vi "SRV_Build Video Stream Rate Command.vi"(10 "Video Stream Rate Period (ms)":u32) -> (1 "Command String":string, 2 "Command Array":u8[](array[numeric]) format="%.0b")   [LabVIEW 2014]
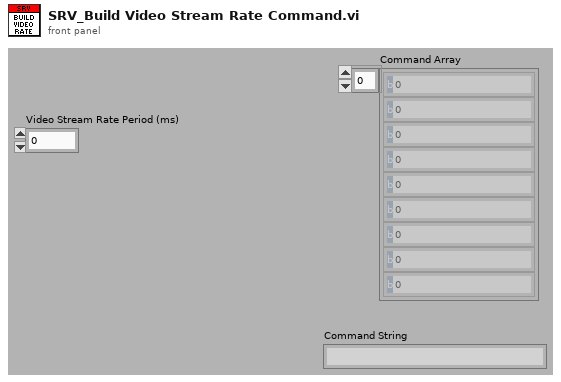
[diagram p1: front panel]
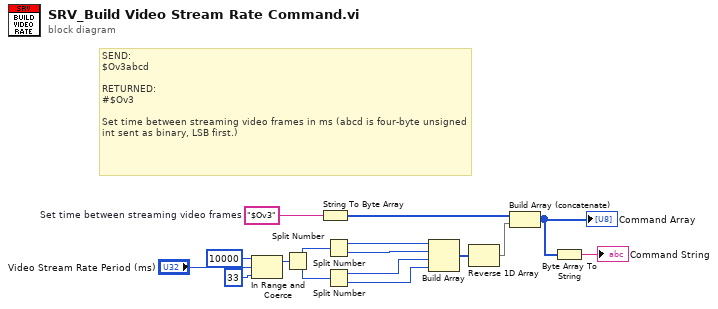
[diagram p0: block diagram]
diagram:
  w6 = "$Ov3"  # Set time between streaming video frames
  # "SEND:\n$Ov3abcd\n\nRETURNED:\n#$Ov3\n\nSet time between streaming video frames in ms (abcd is four-byte unsigned int sent as binary, LSB first.)"
  n1 = In Range and Coerce(upper limit=u32 10000, x="Video Stream Rate Period (ms)", lower limit=u32 33) -> (coerced(x)=w14:u32)  [unwired: 1 out]
  n2 = Split Number(x=w14) -> (hi(x)=w13:u16, lo(x)=w12:u16)
  n3 = String To Byte Array(string=w6) -> (unsigned byte array=w5:u8[])
  n4 = Split Number(x=w13) -> (hi(x)=w11:u8, lo(x)=w10:u8)
  n5 = Split Number(x=w12) -> (hi(x)=w9:u8, lo(x)=w3:u8)
  n6 = Build Array(w11, w10, w9, w3) -> (w7:u8[])
  n7 = Reverse 1D Array(array=w7) -> (reversed array=w4:u8[])
  n8 = Build Array (concatenate)(w5, w4) -> (w2:u8[])
  "Command Array" <- w2
  n9 = Byte Array To String(unsigned byte array=w2) -> (string=→"Command String":string)
